vi "niRFUtil MT UTIL IQ Impairments Frequency Offset.vi"(0 "Waveform In":T1={"x0"=0.0, "dx"=1.0, "y"=[]} caption="input complex waveform" {"y" format="%.2f"; "dx" format="%^.2e"; "x0" format="%^.2e"}, 2 "Frequency Offset, Hz":dbl format="%.2f", 11 "error in (no error)":errorcluster, 13 "Reset? (T)":bool=TRUE) -> (4 "Waveform Out":T1 caption="output complex waveform" {"y" format="%.2f"; "dx" format="%^.2e"; "x0" format="%^.2e"}, 15 "error out":errorcluster)   [LabVIEW 2015, in "niRFUtil.lvlib"]
doc: "Performs the Frequency Offset operation for IQ Impairment of an Input Data Waveform."
uses:
  niRFUtil.lvlib
  Includes/niRFUtil INC Complex Waveform.ctl
  Includes/niRFUtil INC Complex Array.ctl
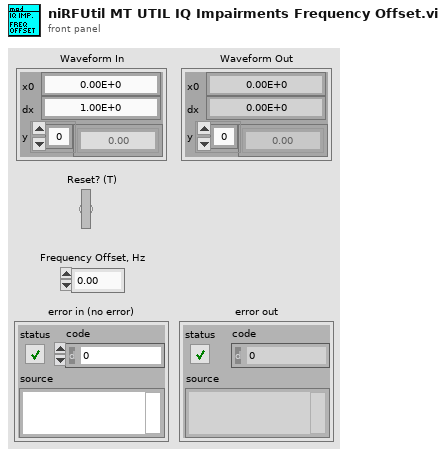
[diagram p1: front panel]
types:
  T1 = typedef "niRFUtil.lvlib/niRFUtil INC Complex Waveform.ctl" = cluster{"x0":dbl, "dx":dbl, "y":T2}
  T2 = typedef "niRFUtil.lvlib/niRFUtil INC Complex Array.ctl" = csg[]
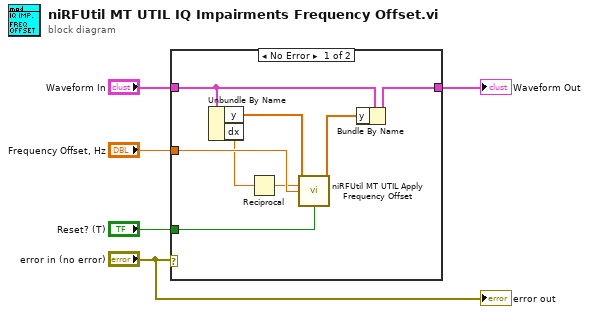
[diagram p0: block diagram]
diagram:
  n1 = case shown="No Error" "error in (no error)" {
    tunnel: "Reset? (T)" -> [w9 _]
    tunnel: "Waveform In" -> [w13 w14]
    tunnel: [w12 w14] -> w2
    tunnel: "Frequency Offset, Hz" -> [w8 _]
    frame No Error {
      n2 = Unbundle By Name(w13) -> ("y"=w10:T2, "dx"=w6:dbl)
      n3 = Reciprocal(x=w6) -> (1/x=w7:dbl)
      n4 = call "niRFUtil MT UTIL Apply Frequency Offset.vi"("Signal In"=w10, "Rate (S/s)"=w7, "Freq Offset (Hz)"=w8, "Reset? (T)"=w9) -> ("Signal Out"=w11:T2)  [unwired: 2 in, 9 out]
      n5 = Bundle By Name(cluster=w13, "y"=w11) -> (w12:T1)
    }
    frame Error {
    }
  }
  "Waveform Out" <- w2
  "error out" <- "error in (no error)"
